vi "Waveform_Append and Sync.vi"(8 "Error":errorcluster, 10 "Waveform To Append":T1, 11 "Waveform":T1) -> (0 "Error Out":errorcluster, 3 "Waveform Out":T1, 5 "Offset Out":i32)   [LabVIEW 2025]
uses:
  Universal Controls/Waveform_Data.ctl
  <vilib>/Waveform/WDTOps.llb/WDT Get Final Time Value DBL.vi
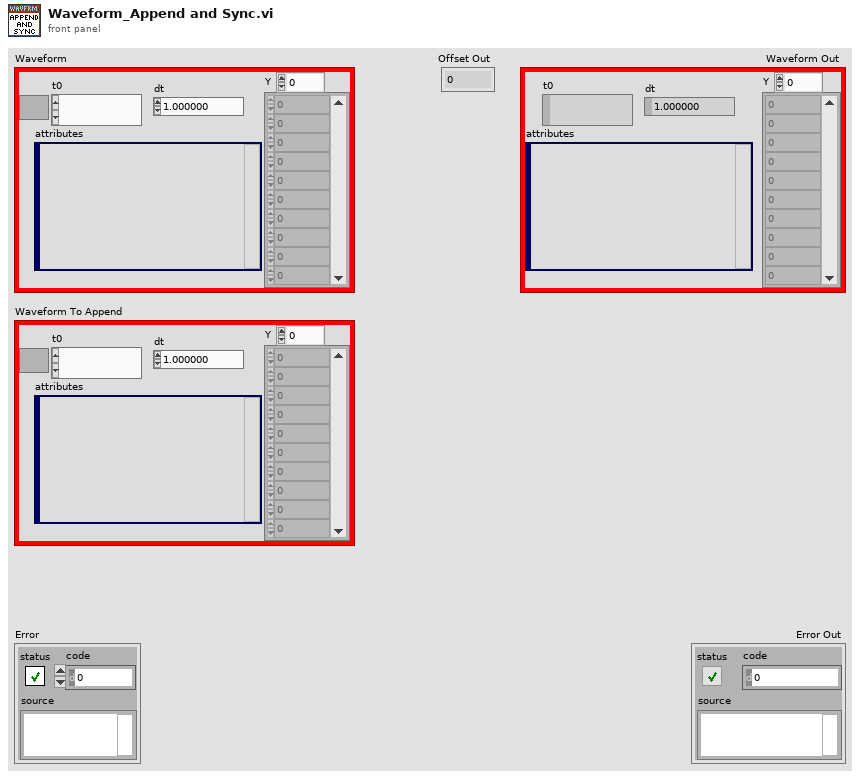
[diagram p1: front panel]
types:
  T1 = typedef "Waveform_Data.ctl" = waveform(dbl)
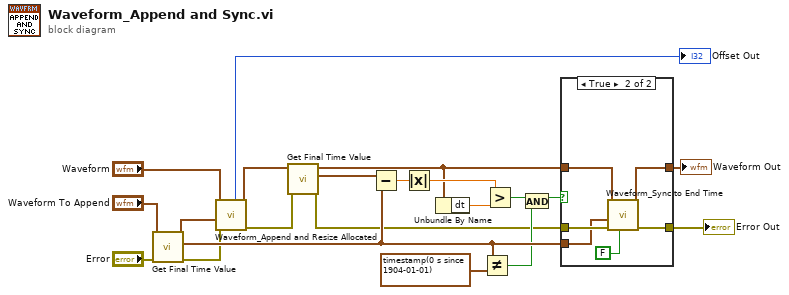
[diagram p0: block diagram]
diagram:
  n1 = call-poly <vilib>:"Get Final Time Value.vi"("error in (no error)"="Error", "waveform in"="Waveform To Append") -> ("error out"=w5:errorcluster, "tf"=w20:timestamp, "waveform out"=w4:waveform(dbl))  [unwired: 7 in]
  n2 = call "Waveform_Append and Resize Allocated.vi"("Error"=w5, "Append"=w4, "Waveform"="Waveform") -> ("Error Out"=w10:errorcluster, "Waveform Out"=w9:T1, "Offset Out"=→"Offset Out":i32)  [unwired: 6 in]
  n3 = call-poly <vilib>:"Get Final Time Value.vi"("error in (no error)"=w10, "waveform in"=w9) -> ("error out"=w11:errorcluster, "tf"=w12:timestamp, "waveform out"=w14:waveform(dbl))  [unwired: 7 in]
  n4 = Subtract(x=w12, y=w20) -> (x-y=w13:dbl)
  n5 = Absolute Value(x=w13) -> (abs(x)=w16:dbl)
  n6 = Unbundle By Name(w14) -> ("dt"=w15:dbl)
  n7 = Not Equal?(x=w20, y=timestamp(0 s since 1904-01-01)) -> (x != y?=w19:bool)
  n8 = Greater?(x=w16, y=w15) -> (0:w17:bool)
  n9 = And(x=w17, y=w19) -> (x .and. y?=w18:bool)
  n10 = case shown="True" w18 {
    tunnel: [w23 w29] -> w6
    tunnel: [w22 w28] -> w7
    tunnel: w11 -> [w22 w27]
    tunnel: w20 -> [_ w26]
    tunnel: w14 -> [w23 w25]
    frame False {
    }
    frame True {
      n11 = call "Waveform_Sync to End Time.vi"("Open(t) Closed(f)"=FALSE, "Error"=w27, "tf"=w26, "Waveform"=w25) -> ("Error Out"=w28:errorcluster, "Waveform Out"=w29:T1)  [unwired: 5 in, 1 out]
    }
  }
  "Error Out" <- w7
  "Waveform Out" <- w6
